vi "JSONRPC-GetNextValue.vi"(7 "unquote strings (false)":bool, 11 "input string":string) -> (2 "after":string, 3 "next":string)   [LabVIEW 2014]
doc: "Search for the next array element in <b>input string</b>."
uses:
  <vilib>/regexp/Match Regular Expression.xnode
panel:
  # "GetNextValue"
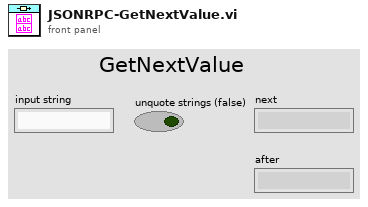
[diagram p1: front panel]
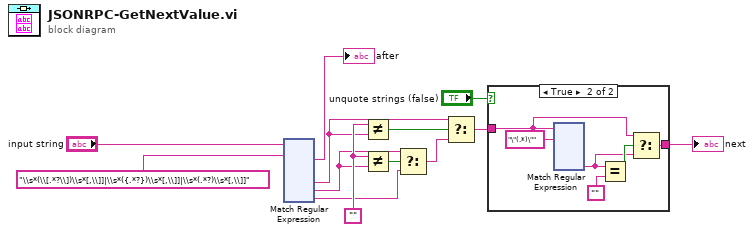
[diagram p0: block diagram]
diagram:
  w8 = ""
  n1 = xnode "Match Regular Expression"("input string"="input string", "regular expression"="\\s*(\\[.*?\\])\\s*[,\\]]|\\s*({.*?})\\s*[,\\]]|\\s*(.*?)\\s*[,\\]]" ("input string")) -> ("after match"=→"after":string, "submatch 1"=w5:string, "submatch 2"=w7:string, "submatch 3"=w1:string)  [unwired: 4 in, 4 out]
  n2 = Not Equal?(x=w8, y=w5) -> (x != y?=w9:bool)
  n3 = Not Equal?(x=w8, y=w7) -> (x != y?=w11:bool)
  n4 = Select(t=w7, s=w11, f=w1) -> (s? t:f=w10:string)
  n5 = Select(t=w5, s=w9, f=w10) -> (s? t:f=w4:string)
  n6 = case shown="True" "unquote strings (false)" {
    tunnel: w4 -> [w14 w15]
    tunnel: [w14 w16] -> w3
    frame False {
    }
    frame True {
      n7 = xnode "Match Regular Expression"("input string"=w15, "regular expression"="\"(.*)\"") -> ("submatch 1"=w17:string)  [unwired: 4 in, 5 out]
      n8 = Equal?(x=w17, y="") -> (x = y?=w18:bool)
      n9 = Select(t=w15, s=w18, f=w17) -> (s? t:f=w16:string)
    }
  }
  "next" <- w3
